vi "hamamatsushowseq.vi"(9 "Enum":enum16{"Get Path", "RunAsync"}(ring)=enum."RunAsync", 11 "Handle in":u32) -> (1 "path":path)   [LabVIEW 2021]
panel:
  in  "Close":bool
  in  "Numeric":u16
  out "Image":T1(plugin-control)
  out "error out":errorcluster
  in  "error in (no error)":errorcluster
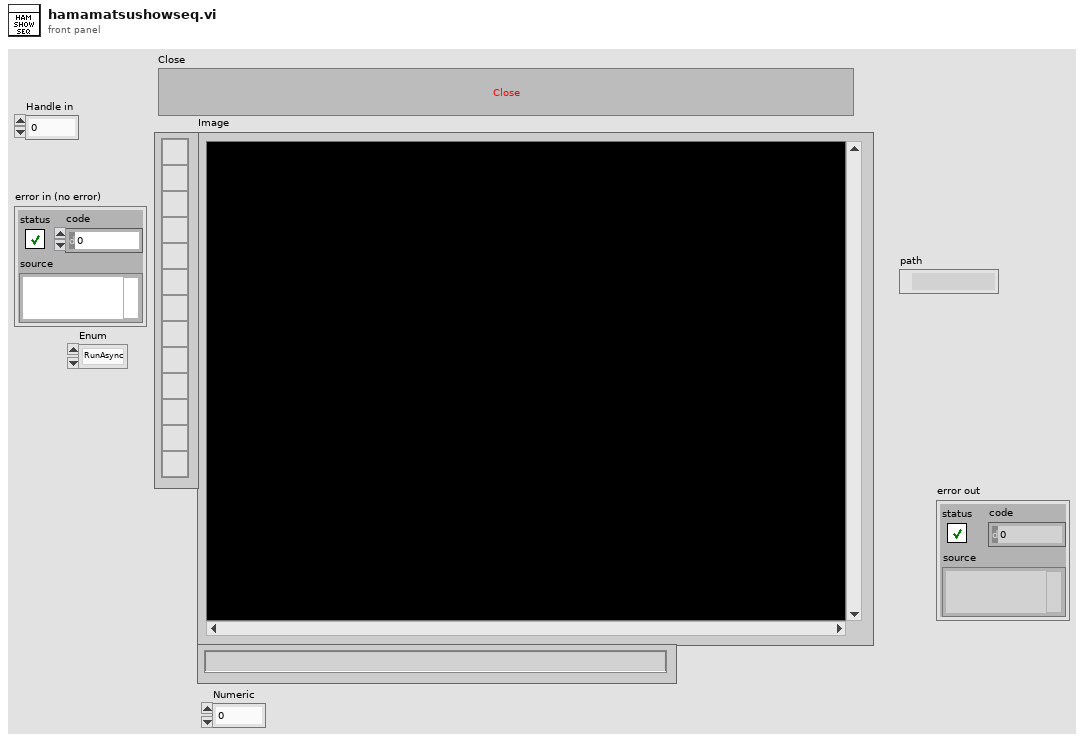
[diagram p1: front panel]
types:
  T1 = typedef "IMAQ Image.ctl" = refnum<image>
  T2 = typedef "Image Type" = u32
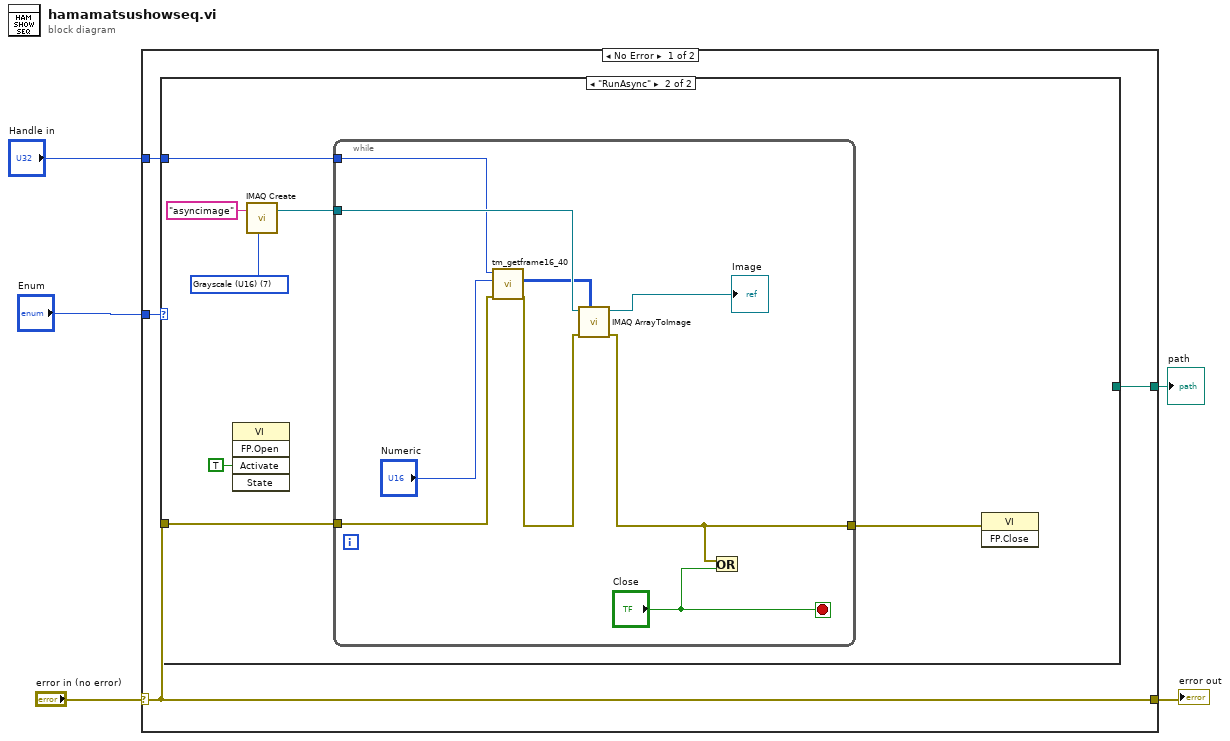
[diagram p0: block diagram]
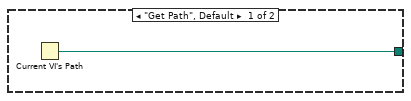
[diagram p2: hidden frame]
diagram:
  n1 = case shown="No Error" "error in (no error)" {
    selector: "error in (no error)" -> [w7 w27]
    tunnel: [w7 w27] -> w2
    tunnel: [w9 _] -> w4
    tunnel: "Enum" -> [w8 _]
    tunnel: "Handle in" -> [w6 _]
    frame No Error {
      n2 = case shown="\"RunAsync\"" w8 {
        tunnel: [w10 _] -> w9
        tunnel: w7 -> [_ w16]
        tunnel: w6 -> [_ w12]
        frame "Get Path", Default {
          n3 = Current VI's Path() -> (path=w10:path)
        }
        frame "RunAsync" {
          w14 = T2 7 items=["Grayscale (U8)", "Grayscale (I16)", "Grayscale (SGL)", "Complex (CSG)", "RGB (U32)", "HSL (U32)", "RGB (U64)", "Grayscale (U16)"] ("Image Type")
          n4 = invoke class="VI" method="FP.Open"("Activate"=TRUE ("Activate?")) -> ()  [unwired: 4 in, 5 out]
          n5 = call "IMAQ Create"("Image Name"="asyncimage", "Image Type"=w14) -> ("New Image"=w15:T1)  [unwired: 3 in, 1 out]
          n6 = while {
            tunnel: w16 -> [w26]
            tunnel: w15 -> [w24]
            tunnel: [w20] -> w11
            tunnel: w12 -> [w18]
            stop <- "Close" stop-if-true
            n7 = call <userlib>:"tm_getframe16_40.vi"("error in (no error)"=w26, "Frame Index"="Numeric", "Handle in"=w18) -> ("error out"=w21:errorcluster, "Data"=w19:u16[][])  [unwired: 5 in, 2 out]
            n8 = call "IMAQ ArrayToImage"("Image Pixels (U16)"=w19, "error in (no error)"=w21, "Image"=w24) -> ("error out"=w20:errorcluster, "Image Out"=→"Image":T1)  [unwired: 7 in]
            n9 = Or(x=w20, y="Close") -> ()  [unwired: 1 out]
          }
          n10 = invoke class="VI" method="FP.Close"(error in=w11) -> ()  [unwired: 2 in, 3 out]
        }
      }
    }
    frame Error {
    }
  }
  "error out" <- w2
  "path" <- w4
